vi "Get Wheels in Steering Frame.vi"   [LabVIEW 2017, in "NI_Robotics_Steering Frame.lvclass"]
doc: "Returns the wheels you specify in <B>steering frame in</B> and properties of those wheels. You must manually select the polymorphic instance to use."
uses:
  <vilib>/robotics/Steering/Steering Frame/NI_Robotics_Steering Frame.lvclass
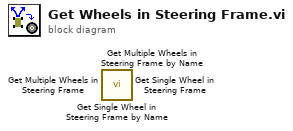
[diagram p0: block diagram]
diagram:
  n1 = call <vilib>:"Get Single Wheel in Steering Frame by Name.vi"() -> ()  [unwired: 5 in, 7 out]
  n2 = call <vilib>:"Get Multiple Wheels in Steering Frame by Name.vi"() -> ()  [unwired: 5 in, 7 out]
  n3 = call <vilib>:"Get Multiple Wheels in Steering Frame.vi"() -> ()  [unwired: 5 in, 7 out]
  n4 = call <vilib>:"Get Single Wheel in Steering Frame.vi"() -> ()  [unwired: 5 in, 7 out]
